vi "CloseRequest.vi"(8 "error in (no error)":errorcluster, 11 "ModuleID":i32) -> (0 "error out":errorcluster)   [LabVIEW 2018, in "AcPwrModule.lvlib"]
doc: "This VI sends a message to close the session(s) to any instrument(s). The intended recipient of the message is Main.vi but any VI with a properly set up event structure can listen for this message and act."
uses:
  AcPwrModule.lvlib
  AcPwrShared/clEventType.ctl
  <vilib>/Utility/error.llb/Error Cluster From Error Code.vi
  <vilib>/ErrorRing/Error Ring.xnode
  AcPwrShared/AcPwrShared.lvlib
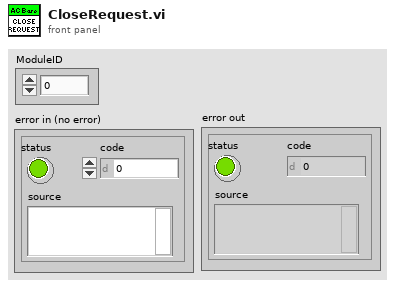
[diagram p1: front panel]
types:
  T1 = typedef "AcPwrShared.lvlib/clRequestEvents.ctl" = cluster{"StopRequest":refnum<user-event>, "PathToINI":refnum<user-event>, " LoadPlugin":refnum<user-event>, "ShowPanel":refnum<user-event>, "PrefDlg":refnum<user-event>, "InitAcPwr":refnum<user-event>, "Reset":refnum<user-event>, "Close":refnum<user-event>, "StopMeas":refnum<user-event>, "StartMeas":refnum<user-event>, "ConfigDevice":refnum<user-event>, "DeviceOn":refnum<user-event>, "DeviceOff":refnum<user-event>, "GetSettings":refnum<user-event>, "SetSettings":refnum<user-event>}
  T2 = typedef "AcPwrShared.lvlib/clEventType.ctl" = cluster{"ModuleID":i32, "Data":variant}
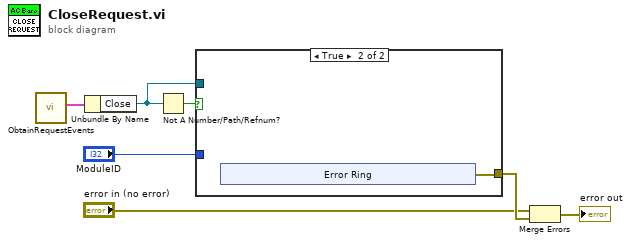
[diagram p0: block diagram]
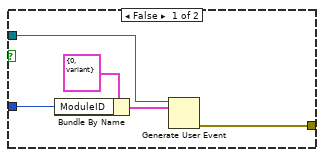
[diagram p2: hidden frame]
diagram:
  n1 = call "ObtainRequestEvents.vi"() -> ("clRequestEvents"=w1:T1)  [unwired: 10 in, 1 out]
  n2 = Unbundle By Name(w1) -> ("Close"=w6:refnum<user-event>)
  n3 = Not A Number/Path/Refnum?(number/path/refnum=w6) -> (NaN/Path/Refnum?=w7:bool)
  n4 = case shown="True" w7 {
    tunnel: w6 -> [w11 _]
    tunnel: "ModuleID" -> [w9 _]
    tunnel: [w10 w13] -> w3
    frame False {
      n5 = Bundle By Name(cluster=T2 {"ModuleID"=0, "Data"=variant} ("clEventType"), "ModuleID"=w9) -> (w12:T2)
      n6 = Generate User Event(user event=w11, event data cluster=w12) -> (error out=w10:errorcluster)  [unwired: 2 in, 1 out]
    }
    frame True {
      n7 = xnode "Error Ring"() -> ("error out"=w13:errorcluster)
    }
  }
  n8 = Merge Errors("error in (no error)", w3) -> (→"error out":errorcluster)
